vi "Path Get SteamLibrary Path.vi"(8 "error in (no error)":errorcluster) -> (0 "error out":errorcluster, 2 "Found":bool, 3 "SteamLibrary Path":path)   [LabVIEW 2018, in "Main Panel.lvlib" / "Main Panel.lvclass"]
uses:
  Main Panel.lvclass
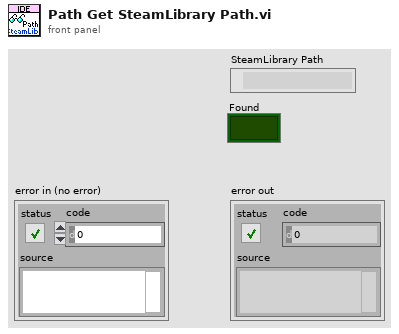
[diagram p1: front panel]
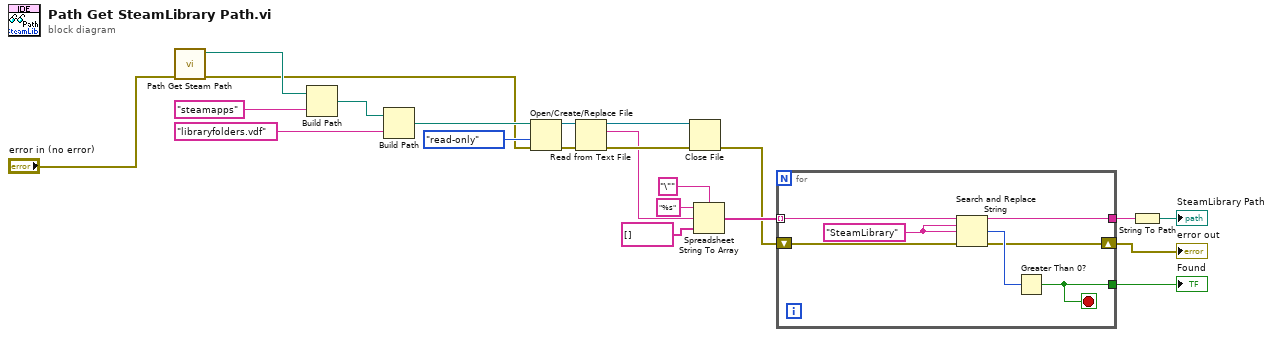
[diagram p0: block diagram]
diagram:
  n1 = call "Path Get Steam Path.vi"("error in (no error)"="error in (no error)") -> ("error out"=w1:errorcluster, "Steam Path"=w3:path)  [unwired: 9 in]
  n2 = Build Path(base path=w3, name or relative path="steamapps") -> (appended path=w21:path)
  n3 = Build Path(base path=w21, name or relative path="libraryfolders.vdf") -> (appended path=w15:path)
  n4 = Open/Create/Replace File(file path (use dialog)=w15, error in=w1, access (0:read/write)=enum16{"read/write", "read-only", "write-only"}."read-only") -> (refnum out=w19:refnum<file>, error out=w18:errorcluster)  [unwired: 3 in, 1 out]
  n5 = Read from Text File(file (use dialog)=w19, error in=w18) -> (refnum out=w17:refnum<file>, text=w13:string, error out=w16:errorcluster)  [unwired: 2 in, 1 out]
  n6 = Close File(refnum=w17, error in=w16) -> (error out=w5:errorcluster)  [unwired: 1 out]
  n7 = Spreadsheet String To Array(delimiter (Tab)="\"" ("element"), format string="%s", spreadsheet string=w13, array type (2D Dbl)=string[] []) -> (array=w10:string[])
  n8 = for {
    tunnel: w10 -> [w28] mode=indexing
    tunnel: [w27] -> w7
    tunnel: [w25] -> w9
    shift-right: [w23] -> w4
    shift-left: w5 -> [w24]
    stop <- w25 stop-if-true
    w29 = "SteamLibrary" ("search string")
    n9 = Search and Replace String(input string=w28, search string=w29, replace string=w29, error in=w24) -> (result string=w27:string, number of replacements=w26:i32, error out=w23:errorcluster)  [unwired: 4 in, 1 out]
    n10 = Greater Than 0?(x=w26) -> (x > 0?=w25:bool)
  }
  "Found" <- w9
  "error out" <- w4
  n11 = String To Path(string=w7) -> (path=→"SteamLibrary Path":path)
